vi "Locate Key.vi"(8 "error in":errorcluster, 9 "key":string, 10 "section":string, 11 "key lookup":variant) -> (0 "error out":errorcluster, 1 "key definition":T1, 2 "found?":bool, 3 "key lookup out":variant)   [LabVIEW 2012, in "configlib.lvlib"]
uses:
  Key Definition.ctl
  configlib.lvlib
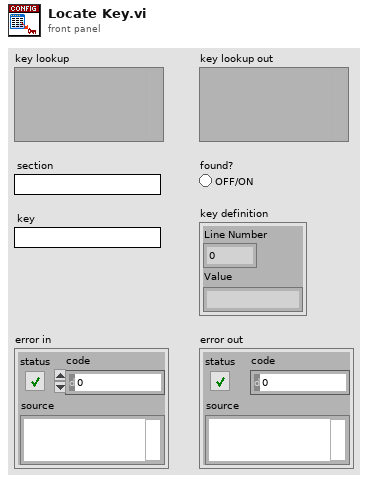
[diagram p1: front panel]
types:
  T1 = typedef "configlib.lvlib/Key Definition.ctl" = cluster{"Line Number":i32, "Value":string}
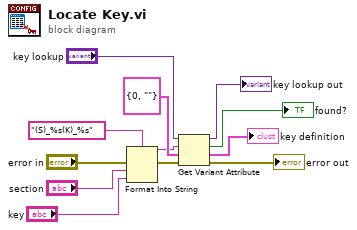
[diagram p0: block diagram]
diagram:
  n1 = Format Into String(format string="(S)_%s(K)_%s", error in="error in", "section", "key") -> (resulting string=w7:string, error out=w6:errorcluster)  [unwired: 1 in]
  n2 = Get Variant Attribute(Variant="key lookup", name=w7, default value (empty Variant)=T1 {"Line Number"=0, "Value"=""} ("Key Definition"), error in=w6) -> (duplicate Variant=→"key lookup out":variant, found=→"found?":bool, value=→"key definition":T1, error out=→"error out":errorcluster)
